vi "Generate Value.vi"(6 "Multiplicador":dbl, 7 "Grandeza":string, 8 "error in (no error)":errorcluster, 9 "Frequencia":dbl, 10 "Valor":dbl, 11 "Calibrator in":refnum<class "Calibrator.lvclass">) -> (0 "error out":errorcluster, 3 "Calibrator out":refnum<class "Calibrator.lvclass">)   [LabVIEW 2015, in "Calibrator.lvclass"]
uses:
  Calibrator.lvclass
  <instrlib>/Fluke 5XXX Series Multicalibrators/Fluke 5XXX Series Multicalibrators.lvlib
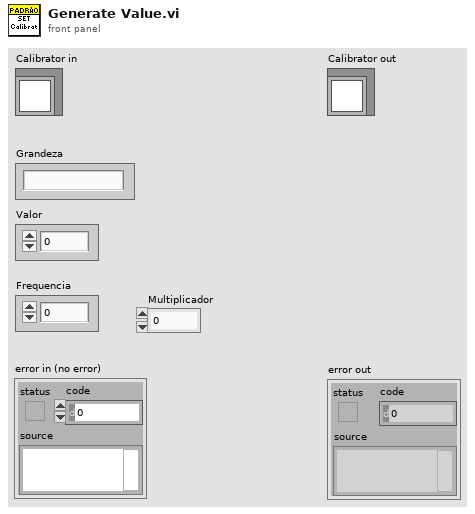
[diagram p1: front panel]
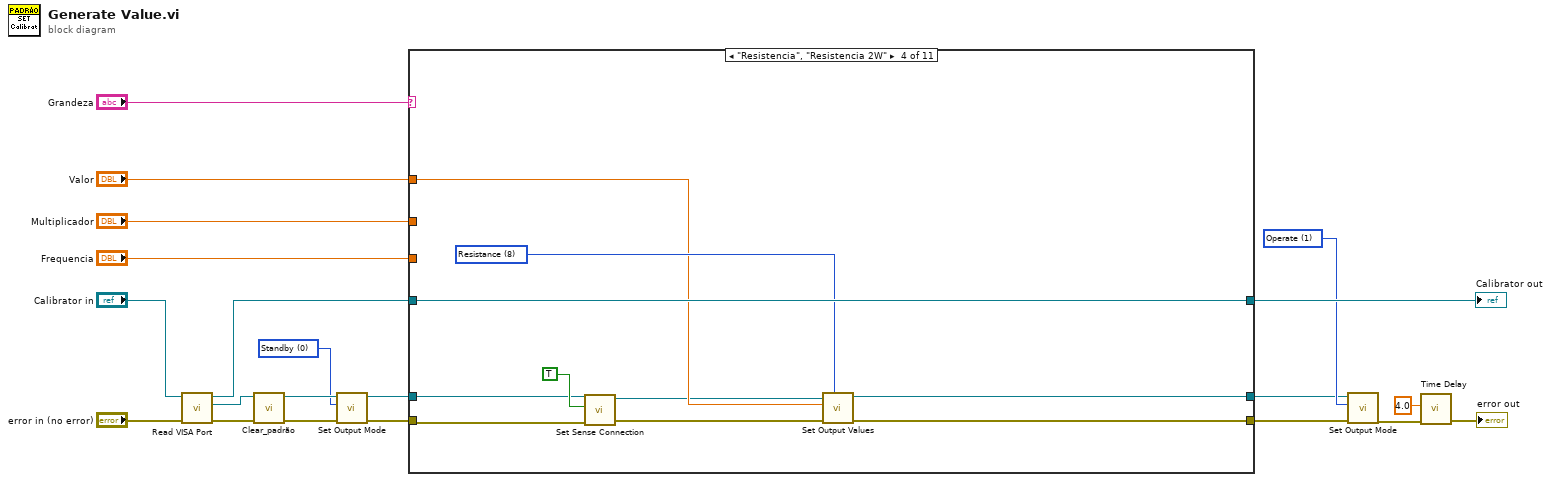
[diagram p0: block diagram]
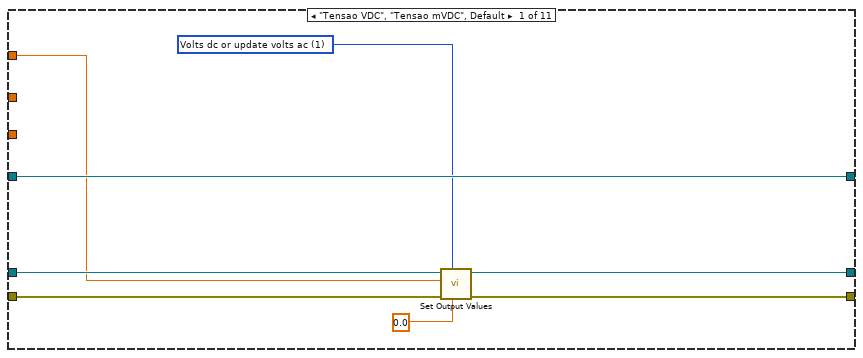
[diagram p2: hidden frame]
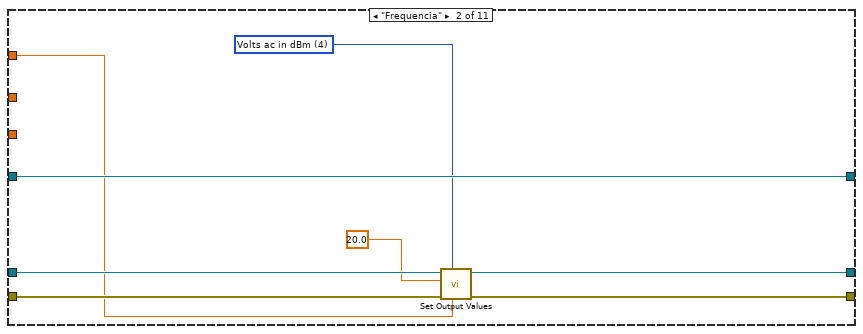
[diagram p3: hidden frame]
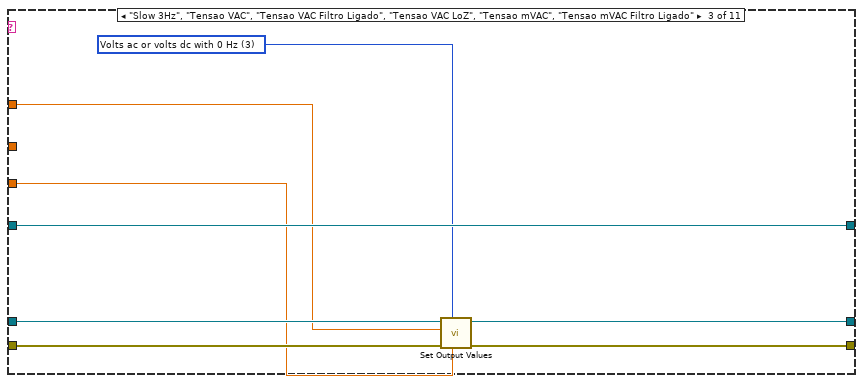
[diagram p4: hidden frame]
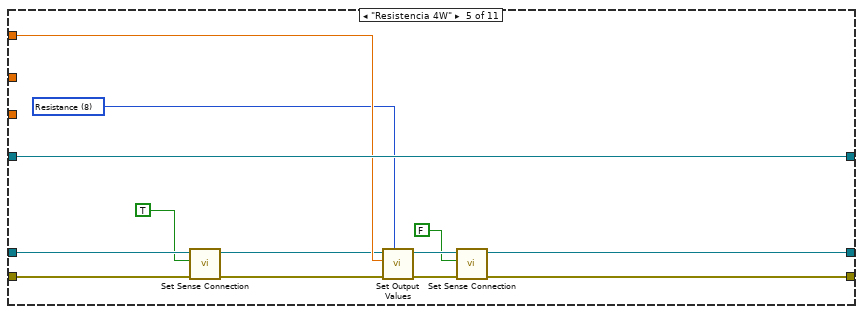
[diagram p5: hidden frame]
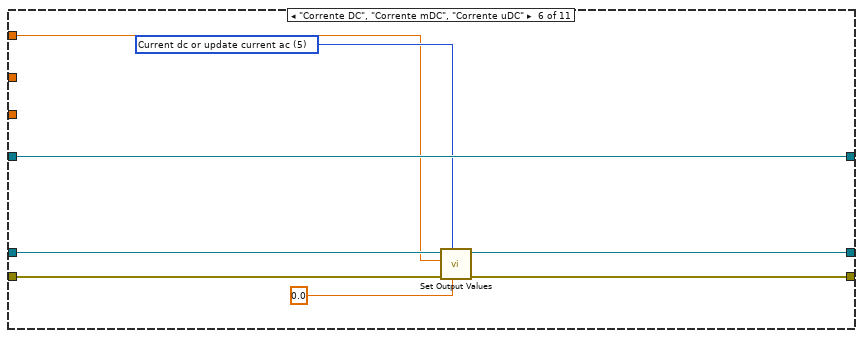
[diagram p6: hidden frame]
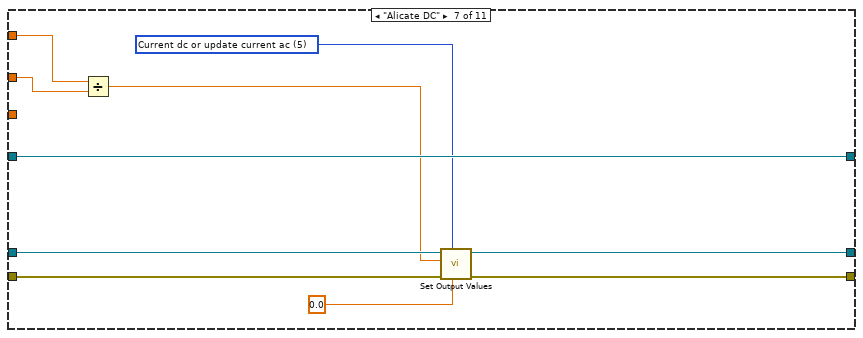
[diagram p7: hidden frame]
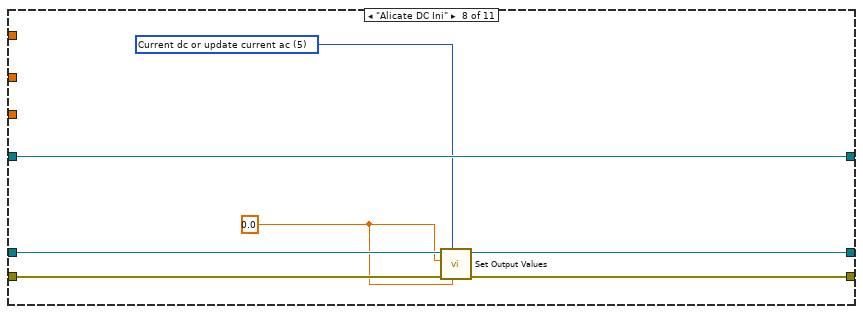
[diagram p8: hidden frame]
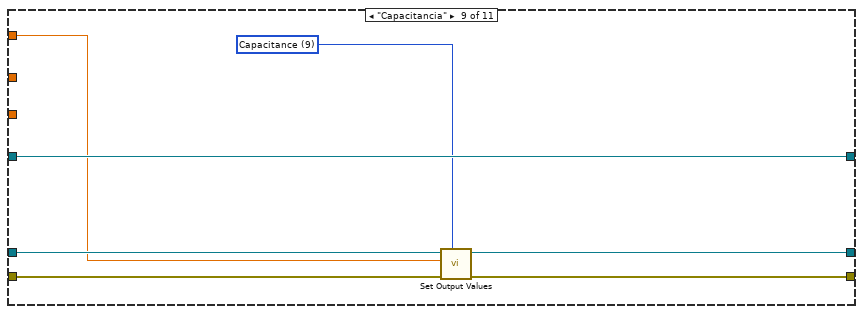
[diagram p9: hidden frame]
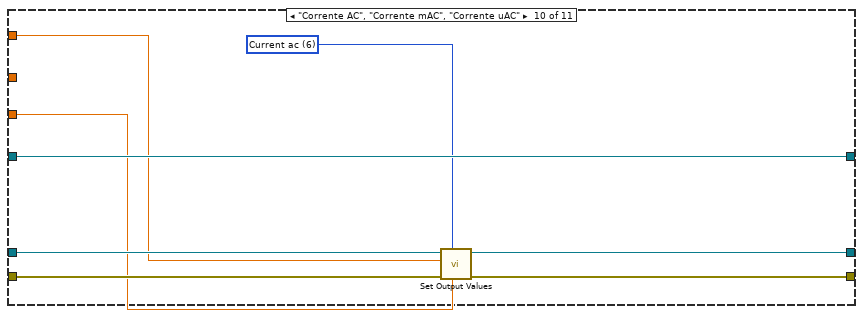
[diagram p10: hidden frame]
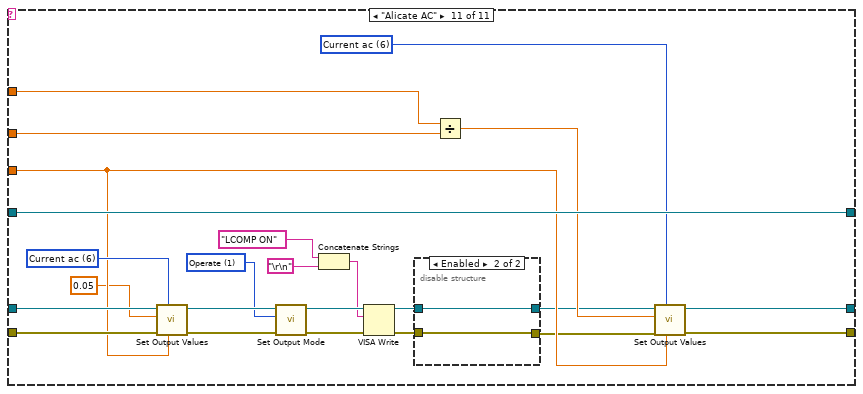
[diagram p11: hidden frame]
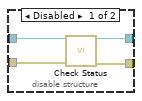
[diagram p12: hidden frame]
diagram:
  w5 = u32 0 items=["Standby", "Operate"] ("Output Mode (0: Standby)")
  w14 = u32 1 items=["Standby", "Operate"] ("Output Mode (0: Standby)")
  n1 = call-dynamic "Read VISA Port.vi"("error in (no error)"="error in (no error)", "Device in"="Calibrator in") -> ("error out"=w10:errorcluster, "VISA Port"=w11:refnum<visa-resource-name>, "Device out"=w18:refnum<class "Calibrator.lvclass">)  [unwired: 7 in]
  n2 = call "Clear_padrão.vi"("error in (no error)"=w10, "VISA resource name"=w11) -> ("error out"=w7:errorcluster, "VISA resource name out"=w6:refnum<visa-resource-name>)  [unwired: 8 in]
  n3 = call <instrlib>:"Set Output Mode.vi"("error in (no error)"=w7, "Output Mode (0: Standby)"=w5, "VISA resource name"=w6) -> ("error out"=w8:errorcluster, "VISA resource name out"=w9:refnum<visa-resource-name>)  [unwired: 7 in]
  n4 = case shown="\"Resistencia\", \"Resistencia 2W\"" "Grandeza" {
    tunnel: [w27 w35 w43 w53 w64 w74 w84 w91 w98 w106 w130] -> w12
    tunnel: [w29 w37 w45 w55 w68 w76 w86 w93 w100 w108 w132] -> w21
    tunnel: w18 -> [w29 w37 w45 w55 w68 w76 w86 w93 w100 w108 w132]
    tunnel: w9 -> [w25 w33 w41 w49 w61 w72 w82 w89 w96 w104 w122]
    tunnel: w8 -> [w26 w34 w42 w48 w59 w73 w83 w90 w97 w105 w123]
    tunnel: "Valor" -> [w23 w31 w40 w52 w67 w71 w78 _ w95 w103 w128]
    tunnel: "Frequencia" -> [_ _ w39 _ _ _ _ _ _ w101 w120]
    tunnel: [w22 w32 w38 w51 w63 w70 w81 w88 w94 w102 w129] -> w13
    tunnel: "Multiplicador" -> [_ _ _ _ _ _ w77 _ _ _ w127]
    frame "Tensao VDC", "Tensao mVDC", Default {
      w28 = u32 1 items=["Amplitude", "Volts dc or update volts ac", "Volts ac dBm update", "Volts ac or volts dc with 0 Hz", "Volts ac in dBm", "Current dc or update current ac", "Current ac", "Update frequency", "Resistance", "Capacitance", "Temperature (Celsius)", "Temperature (Fahrenheit)", "Power dc or update power ac", "Power ac", "Dual volts dc or update dual ac", "Dual volts ac in volts", "Power ac in dBm update", "Power ac in dBm", "Dual volts ac in dBm update", "Dual volts ac in dBm"] ("Output Value(s) (0 - Amplitude)")
      n5 = call <instrlib>:"Set Output Values.vi"("Fundamental Frequency (0.0 Hz)"=0.0, "Output Value(s) (0 - Amplitude)"=w28, "error in (no error)"=w26, "Primary Value (0.0)"=w23, "VISA resource name"=w25) -> ("error out"=w27:errorcluster, "VISA resource name out"=w22:refnum<visa-resource-name>)  [unwired: 5 in]
    }
    frame "Frequencia" {
      w36 = u32 4 items=["Amplitude", "Volts dc or update volts ac", "Volts ac dBm update", "Volts ac or volts dc with 0 Hz", "Volts ac in dBm", "Current dc or update current ac", "Current ac", "Update frequency", "Resistance", "Capacitance", "Temperature (Celsius)", "Temperature (Fahrenheit)", "Power dc or update power ac", "Power ac", "Dual volts dc or update dual ac", "Dual volts ac in volts", "Power ac in dBm update", "Power ac in dBm", "Dual volts ac in dBm update", "Dual volts ac in dBm"] ("Output Value(s) (0 - Amplitude)")
      n6 = call <instrlib>:"Set Output Values.vi"("Fundamental Frequency (0.0 Hz)"=w31, "Output Value(s) (0 - Amplitude)"=w36, "error in (no error)"=w34, "Primary Value (0.0)"=20.0, "VISA resource name"=w33) -> ("error out"=w35:errorcluster, "VISA resource name out"=w32:refnum<visa-resource-name>)  [unwired: 5 in]
    }
    frame "Slow 3Hz", "Tensao VAC", "Tensao VAC Filtro Ligado", "Tensao VAC LoZ", "Tensao mVAC", "Tensao mVAC Filtro Ligado" {
      w44 = u32 3 items=["Amplitude", "Volts dc or update volts ac", "Volts ac dBm update", "Volts ac or volts dc with 0 Hz", "Volts ac in dBm", "Current dc or update current ac", "Current ac", "Update frequency", "Resistance", "Capacitance", "Temperature (Celsius)", "Temperature (Fahrenheit)", "Power dc or update power ac", "Power ac", "Dual volts dc or update dual ac", "Dual volts ac in volts", "Power ac in dBm update", "Power ac in dBm", "Dual volts ac in dBm update", "Dual volts ac in dBm"] ("Output Value(s) (0 - Amplitude)")
      n7 = call <instrlib>:"Set Output Values.vi"("Fundamental Frequency (0.0 Hz)"=w39, "Output Value(s) (0 - Amplitude)"=w44, "error in (no error)"=w42, "Primary Value (0.0)"=w40, "VISA resource name"=w41) -> ("error out"=w43:errorcluster, "VISA resource name out"=w38:refnum<visa-resource-name>)  [unwired: 5 in]
    }
    frame "Resistencia", "Resistencia 2W" {
      w54 = u32 8 items=["Amplitude", "Volts dc or update volts ac", "Volts ac dBm update", "Volts ac or volts dc with 0 Hz", "Volts ac in dBm", "Current dc or update current ac", "Current ac", "Update frequency", "Resistance", "Capacitance", "Temperature (Celsius)", "Temperature (Fahrenheit)", "Power dc or update power ac", "Power ac", "Dual volts dc or update dual ac", "Dual volts ac in volts", "Power ac in dBm update", "Power ac in dBm", "Dual volts ac in dBm update", "Dual volts ac in dBm"] ("Output Value(s) (0 - Amplitude)")
      n8 = call <instrlib>:"Set Sense Connection.vi"("error in (no error)"=w48, "Sense Connection (T: Internal)"=TRUE, "VISA resource name"=w49) -> ("error out"=w46:errorcluster, "VISA resource name out"=w47:refnum<visa-resource-name>)  [unwired: 7 in]
      n9 = call <instrlib>:"Set Output Values.vi"("Output Value(s) (0 - Amplitude)"=w54, "error in (no error)"=w46, "Primary Value (0.0)"=w52, "VISA resource name"=w47) -> ("error out"=w53:errorcluster, "VISA resource name out"=w51:refnum<visa-resource-name>)  [unwired: 6 in]
    }
    frame "Resistencia 4W" {
      w60 = u32 8 items=["Amplitude", "Volts dc or update volts ac", "Volts ac dBm update", "Volts ac or volts dc with 0 Hz", "Volts ac in dBm", "Current dc or update current ac", "Current ac", "Update frequency", "Resistance", "Capacitance", "Temperature (Celsius)", "Temperature (Fahrenheit)", "Power dc or update power ac", "Power ac", "Dual volts dc or update dual ac", "Dual volts ac in volts", "Power ac in dBm update", "Power ac in dBm", "Dual volts ac in dBm update", "Dual volts ac in dBm"] ("Output Value(s) (0 - Amplitude)")
      n10 = call <instrlib>:"Set Sense Connection.vi"("error in (no error)"=w59, "Sense Connection (T: Internal)"=TRUE, "VISA resource name"=w61) -> ("error out"=w56:errorcluster, "VISA resource name out"=w57:refnum<visa-resource-name>)  [unwired: 7 in]
      n11 = call <instrlib>:"Set Output Values.vi"("Output Value(s) (0 - Amplitude)"=w60, "error in (no error)"=w56, "Primary Value (0.0)"=w67, "VISA resource name"=w57) -> ("error out"=w65:errorcluster, "VISA resource name out"=w66:refnum<visa-resource-name>)  [unwired: 6 in]
      n12 = call <instrlib>:"Set Sense Connection.vi"("error in (no error)"=w65, "Sense Connection (T: Internal)"=FALSE, "VISA resource name"=w66) -> ("error out"=w64:errorcluster, "VISA resource name out"=w63:refnum<visa-resource-name>)  [unwired: 7 in]
    }
    frame "Corrente DC", "Corrente mDC", "Corrente uDC" {
      w75 = u32 5 items=["Amplitude", "Volts dc or update volts ac", "Volts ac dBm update", "Volts ac or volts dc with 0 Hz", "Volts ac in dBm", "Current dc or update current ac", "Current ac", "Update frequency", "Resistance", "Capacitance", "Temperature (Celsius)", "Temperature (Fahrenheit)", "Power dc or update power ac", "Power ac", "Dual volts dc or update dual ac", "Dual volts ac in volts", "Power ac in dBm update", "Power ac in dBm", "Dual volts ac in dBm update", "Dual volts ac in dBm"] ("Output Value(s) (0 - Amplitude)")
      n13 = call <instrlib>:"Set Output Values.vi"("Fundamental Frequency (0.0 Hz)"=0.0, "Output Value(s) (0 - Amplitude)"=w75, "error in (no error)"=w73, "Primary Value (0.0)"=w71, "VISA resource name"=w72) -> ("error out"=w74:errorcluster, "VISA resource name out"=w70:refnum<visa-resource-name>)  [unwired: 5 in]
    }
    frame "Alicate DC" {
      w85 = u32 5 items=["Amplitude", "Volts dc or update volts ac", "Volts ac dBm update", "Volts ac or volts dc with 0 Hz", "Volts ac in dBm", "Current dc or update current ac", "Current ac", "Update frequency", "Resistance", "Capacitance", "Temperature (Celsius)", "Temperature (Fahrenheit)", "Power dc or update power ac", "Power ac", "Dual volts dc or update dual ac", "Dual volts ac in volts", "Power ac in dBm update", "Power ac in dBm", "Dual volts ac in dBm update", "Dual volts ac in dBm"] ("Output Value(s) (0 - Amplitude)")
      n14 = Divide(x=w78, y=w77) -> (x/y=w79:dbl)
      n15 = call <instrlib>:"Set Output Values.vi"("Fundamental Frequency (0.0 Hz)"=0.0, "Output Value(s) (0 - Amplitude)"=w85, "error in (no error)"=w83, "Primary Value (0.0)"=w79, "VISA resource name"=w82) -> ("error out"=w84:errorcluster, "VISA resource name out"=w81:refnum<visa-resource-name>)  [unwired: 5 in]
    }
    frame "Alicate DC Ini" {
      w87 = 0.0 ("Fundamental Frequency (0.0 Hz)")
      w92 = u32 5 items=["Amplitude", "Volts dc or update volts ac", "Volts ac dBm update", "Volts ac or volts dc with 0 Hz", "Volts ac in dBm", "Current dc or update current ac", "Current ac", "Update frequency", "Resistance", "Capacitance", "Temperature (Celsius)", "Temperature (Fahrenheit)", "Power dc or update power ac", "Power ac", "Dual volts dc or update dual ac", "Dual volts ac in volts", "Power ac in dBm update", "Power ac in dBm", "Dual volts ac in dBm update", "Dual volts ac in dBm"] ("Output Value(s) (0 - Amplitude)")
      n16 = call <instrlib>:"Set Output Values.vi"("Fundamental Frequency (0.0 Hz)"=w87, "Output Value(s) (0 - Amplitude)"=w92, "error in (no error)"=w90, "Primary Value (0.0)"=w87, "VISA resource name"=w89) -> ("error out"=w91:errorcluster, "VISA resource name out"=w88:refnum<visa-resource-name>)  [unwired: 5 in]
    }
    frame "Capacitancia" {
      w99 = u32 9 items=["Amplitude", "Volts dc or update volts ac", "Volts ac dBm update", "Volts ac or volts dc with 0 Hz", "Volts ac in dBm", "Current dc or update current ac", "Current ac", "Update frequency", "Resistance", "Capacitance", "Temperature (Celsius)", "Temperature (Fahrenheit)", "Power dc or update power ac", "Power ac", "Dual volts dc or update dual ac", "Dual volts ac in volts", "Power ac in dBm update", "Power ac in dBm", "Dual volts ac in dBm update", "Dual volts ac in dBm"] ("Output Value(s) (0 - Amplitude)")
      n17 = call <instrlib>:"Set Output Values.vi"("Output Value(s) (0 - Amplitude)"=w99, "error in (no error)"=w97, "Primary Value (0.0)"=w95, "VISA resource name"=w96) -> ("error out"=w98:errorcluster, "VISA resource name out"=w94:refnum<visa-resource-name>)  [unwired: 6 in]
    }
    frame "Corrente AC", "Corrente mAC", "Corrente uAC" {
      w107 = u32 6 items=["Amplitude", "Volts dc or update volts ac", "Volts ac dBm update", "Volts ac or volts dc with 0 Hz", "Volts ac in dBm", "Current dc or update current ac", "Current ac", "Update frequency", "Resistance", "Capacitance", "Temperature (Celsius)", "Temperature (Fahrenheit)", "Power dc or update power ac", "Power ac", "Dual volts dc or update dual ac", "Dual volts ac in volts", "Power ac in dBm update", "Power ac in dBm", "Dual volts ac in dBm update", "Dual volts ac in dBm"] ("Output Value(s) (0 - Amplitude)")
      n18 = call <instrlib>:"Set Output Values.vi"("Fundamental Frequency (0.0 Hz)"=w101, "Output Value(s) (0 - Amplitude)"=w107, "error in (no error)"=w105, "Primary Value (0.0)"=w103, "VISA resource name"=w104) -> ("error out"=w106:errorcluster, "VISA resource name out"=w102:refnum<visa-resource-name>)  [unwired: 5 in]
    }
    frame "Alicate AC" {
      w116 = u32 1 items=["Standby", "Operate"] ("Output Mode (0: Standby)")
      w121 = u32 6 items=["Amplitude", "Volts dc or update volts ac", "Volts ac dBm update", "Volts ac or volts dc with 0 Hz", "Volts ac in dBm", "Current dc or update current ac", "Current ac", "Update frequency", "Resistance", "Capacitance", "Temperature (Celsius)", "Temperature (Fahrenheit)", "Power dc or update power ac", "Power ac", "Dual volts dc or update dual ac", "Dual volts ac in volts", "Power ac in dBm update", "Power ac in dBm", "Dual volts ac in dBm update", "Dual volts ac in dBm"] ("Output Value(s) (0 - Amplitude)")
      w131 = u32 6 items=["Amplitude", "Volts dc or update volts ac", "Volts ac dBm update", "Volts ac or volts dc with 0 Hz", "Volts ac in dBm", "Current dc or update current ac", "Current ac", "Update frequency", "Resistance", "Capacitance", "Temperature (Celsius)", "Temperature (Fahrenheit)", "Power dc or update power ac", "Power ac", "Dual volts dc or update dual ac", "Dual volts ac in volts", "Power ac in dBm update", "Power ac in dBm", "Dual volts ac in dBm update", "Dual volts ac in dBm"] ("Output Value(s) (0 - Amplitude)")
      n19 = call <instrlib>:"Set Output Values.vi"("Fundamental Frequency (0.0 Hz)"=w120, "Output Value(s) (0 - Amplitude)"=w121, "error in (no error)"=w123, "Primary Value (0.0)"=0.05, "VISA resource name"=w122) -> ("error out"=w118:errorcluster, "VISA resource name out"=w117:refnum<visa-resource-name>)  [unwired: 5 in]
      n20 = call <instrlib>:"Set Output Mode.vi"("error in (no error)"=w118, "Output Mode (0: Standby)"=w116, "VISA resource name"=w117) -> ("error out"=w114:errorcluster, "VISA resource name out"=w115:refnum<visa-resource-name>)  [unwired: 7 in]
      n21 = Concatenate Strings("LCOMP ON" ("Reset Command"), "\r\n") -> (w110:string)
      n22 = VISA Write(VISA resource name=w115, write buffer=w110, error in (no error)=w114) -> (VISA resource name out=w124:refnum<visa-resource-name>, error out=w125:errorcluster)  [unwired: 1 out]
      n23 = disable-structure shown="Enabled" {
        disable-tunnel: w125 -> [w136 w137]
        disable-tunnel: w124 -> [w135 w138]
        disable-tunnel: [w134 w137] -> w113
        disable-tunnel: [w133 w138] -> w112
        frame Disabled {
          n24 = call <instrlib>:"Check Status.vi"("VISA resource name"=w135, "error in (no error)"=w136) -> ("VISA resource name out"=w133:refnum<visa-resource-name>, "error out"=w134:errorcluster)  [unwired: 12 in]
        }
        frame Enabled {
        }
      }
      n25 = Divide(x=w128, y=w127) -> (x/y=w126:dbl)
      n26 = call <instrlib>:"Set Output Values.vi"("Fundamental Frequency (0.0 Hz)"=w120, "Output Value(s) (0 - Amplitude)"=w131, "error in (no error)"=w113, "Primary Value (0.0)"=w126, "VISA resource name"=w112) -> ("error out"=w130:errorcluster, "VISA resource name out"=w129:refnum<visa-resource-name>)  [unwired: 5 in]
    }
  }
  "Calibrator out" <- w21
  n27 = call <instrlib>:"Set Output Mode.vi"("error in (no error)"=w12, "Output Mode (0: Standby)"=w14, "VISA resource name"=w13) -> ("error out"=w3:errorcluster)  [unwired: 7 in, 1 out]
  n28 = call "Time Delay"("error in (no error)"=w3, "Delay Time (s)"=4.0) -> ("error out"=→"error out":errorcluster)  [unwired: 9 in]
